vi "create_file.vi"(8 "error in (no error)":errorcluster) -> (0 "error out":errorcluster, 3 "appended path":path)   [LabVIEW 2020]
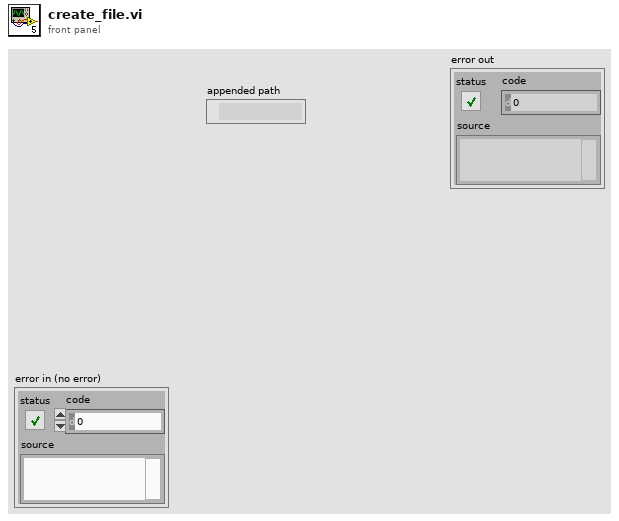
[diagram p1: front panel]
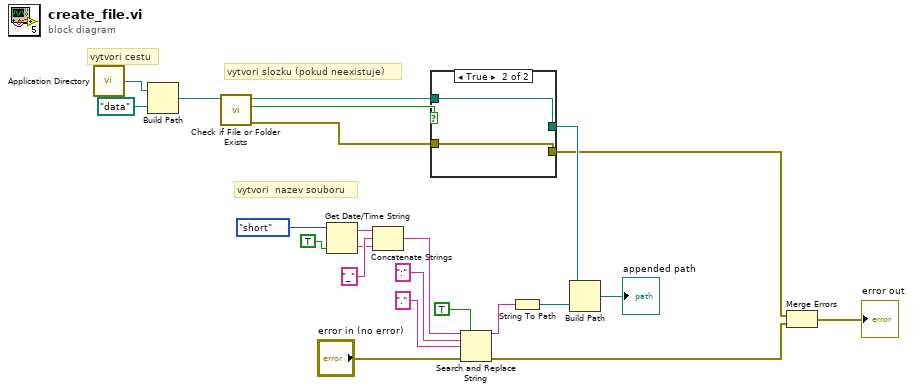
[diagram p0: block diagram]
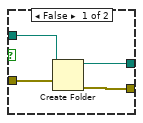
[diagram p2: hidden frame]
diagram:
  # "vytvori  nazev souboru"
  # "vytvori cestu"
  # "vytvori slozku (pokud neexistuje)"
  n1 = call <vilib>:"Application Directory.vi"() -> ("Application Directory"=w21:path)
  n2 = Build Path(base path=w21, name or relative path=path "data" ("path")) -> (appended path=w19:path)
  n3 = call <vilib>:"Check if File or Folder Exists.vi"("path"=w19) -> ("error out"=w7:errorcluster, "file or folder exists?"=w5:bool, "dup path"=w4:path)  [unwired: 8 in]
  n4 = Get Date/Time String(date format (0)=enum16{"short", "long", "abbreviated"}."short", want seconds? (F)=TRUE) -> (date string=w8:string, time string=w15:string)  [unwired: 1 in]
  n5 = Concatenate Strings(w8, "_" ("string"), w15) -> (w10:string)
  n6 = case shown="True" w5 {
    tunnel: w7 -> [w27 w29]
    tunnel: [w26 w29] -> w3
    tunnel: [w25 w28] -> w6
    tunnel: w4 -> [w24 w28]
    frame False {
      n7 = Create Folder(path (use dialog)=w24, error in=w27) -> (created path=w25:path, error out=w26:errorcluster)  [unwired: 1 in, 1 out]
    }
    frame True {
    }
  }
  n8 = Search and Replace String(replace all?=TRUE ("replace all? (F)"), input string=w10, search string=":", replace string="." ("replace string (\"\")"), error in="error in (no error)") -> (result string=w14:string, error out=w2:errorcluster)  [unwired: 3 in, 2 out]
  n9 = String To Path(string=w14) -> (path=w23:path)
  n10 = Build Path(base path=w6, name or relative path=w23) -> (appended path=→"appended path":path)
  n11 = Merge Errors(w3, w2) -> (→"error out":errorcluster)
